vi "HEWH ANSI Display.vi"(5 "Calculation Type":string(combo), 7 "Stop Timer":dbl=1200.0 format="%#_13g", 8 "Error In":errorcluster, 9 "Software Elapsed Time":dbl, 11 "ANSI Rate In":T1) -> (0 "Error Out":errorcluster, 1 "Raw Timer":dbl, 2 "ANSI Display":string, 3 "ANSI Rate Out":T1)   [LabVIEW 2023]
uses:
  HEWH ANSI Rate.ctl
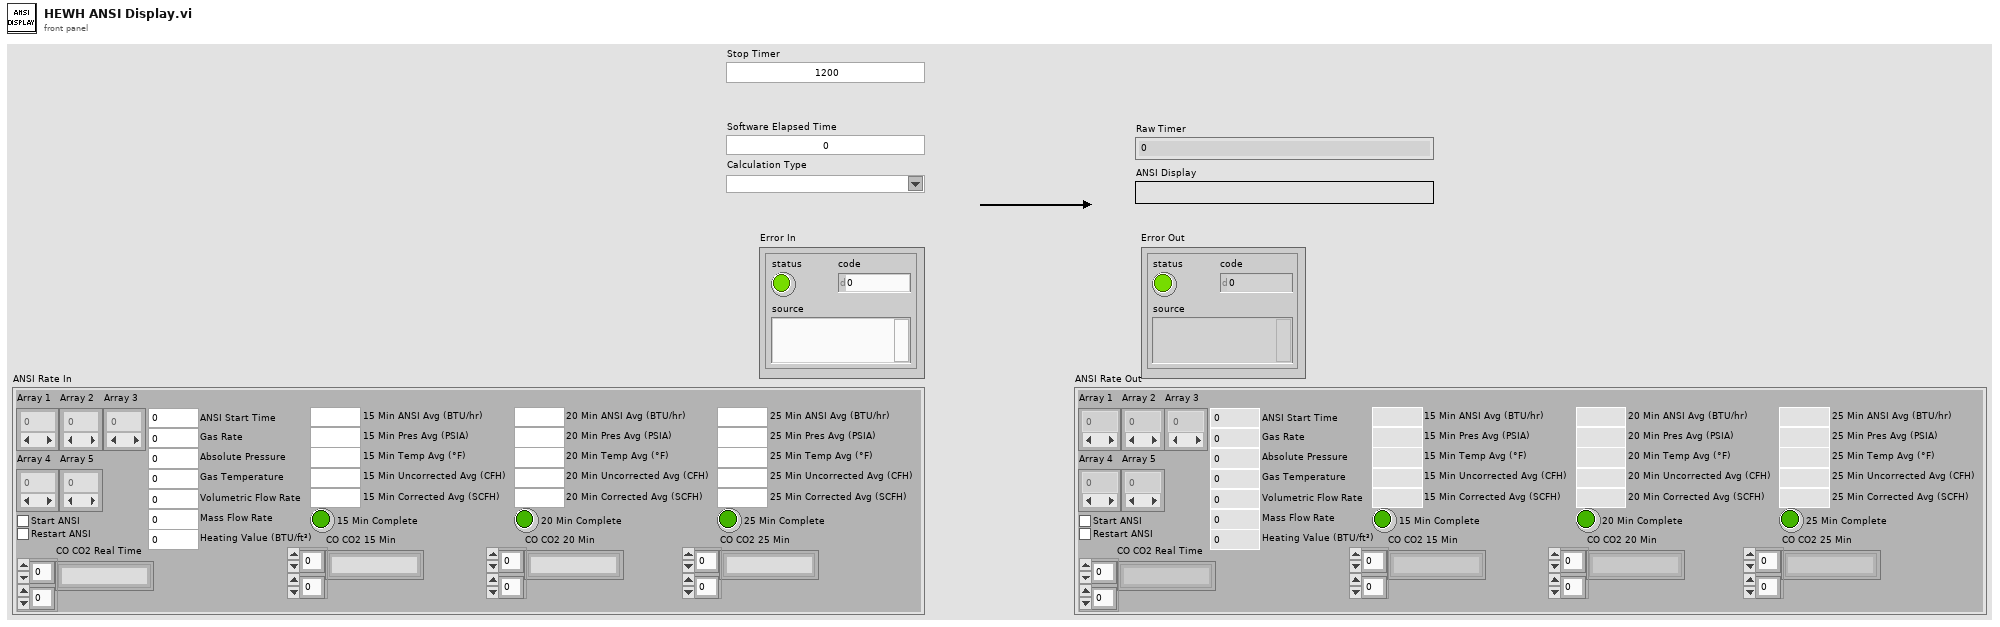
[diagram p1: front panel]
types:
  T1 = typedef "HEWH ANSI Rate.ctl" = cluster{"Array 1":dbl[], "Array 3":dbl[], "Array 2":dbl[], "Start ANSI":bool, "ANSI Start Time":dbl, "Restart ANSI":bool, "15 Min ANSI Avg (BTU/hr)":dbl, "20 Min ANSI Avg (BTU/hr)":dbl, "25 Min ANSI Avg (BTU/hr)":dbl, "Absolute Pressure":dbl, "Gas Temperature":dbl, "Volumetric Flow Rate":dbl, "Mass Flow Rate":dbl, "Array 4":dbl[], "Array 5":dbl[], "Gas Rate":dbl, "15 Min Pres Avg (PSIA)":dbl, "20 Min Pres Avg (PSIA)":dbl, "25 Min Pres Avg (PSIA)":dbl, "15 Min Temp Avg (°F) ":dbl, "20 Min Temp Avg (°F)":dbl, "25 Min Temp Avg (°F)":dbl, "15 Min Uncorrected Avg (CFH)":dbl, "20 Min Uncorrected Avg (CFH)":dbl, "25 Min Uncorrected Avg (CFH)":dbl, "15 Min Corrected Avg (SCFH)":dbl, "20 Min Corrected Avg (SCFH)":dbl, "25 Min Corrected Avg (SCFH)":dbl, "15 Min Complete":bool, "20 Min Complete":bool, "25 Min Complete":bool, "Heating Value (BTU/ft³)":dbl, "CO CO2 15 Min":string[][], "CO CO2 20 Min":string[][], "CO CO2 25 Min":string[][], "CO CO2 Real Time":string[][]}
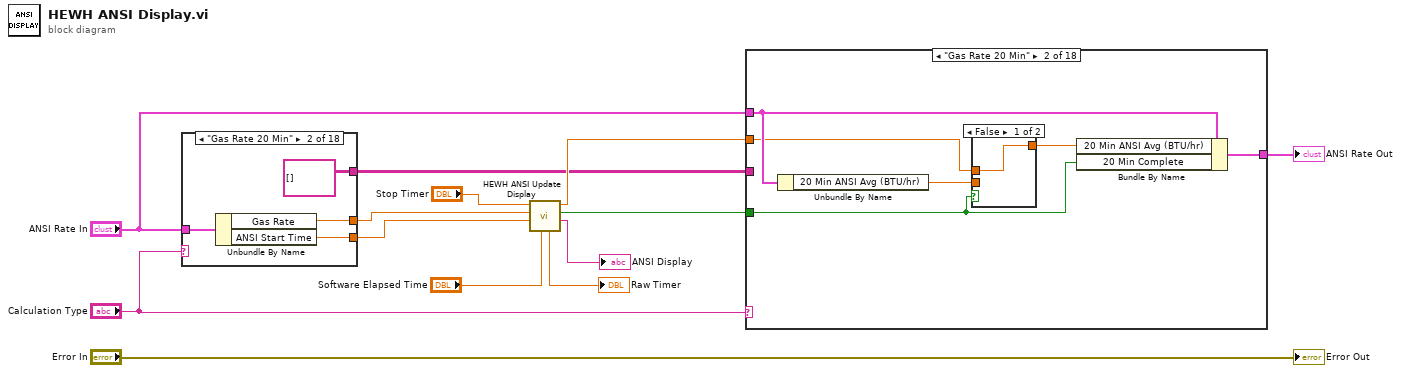
[diagram p0: block diagram]
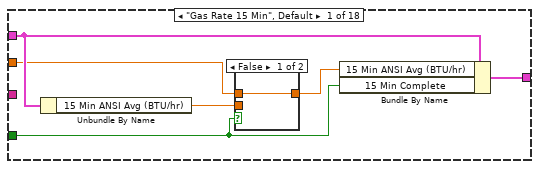
[diagram p2: hidden frame]
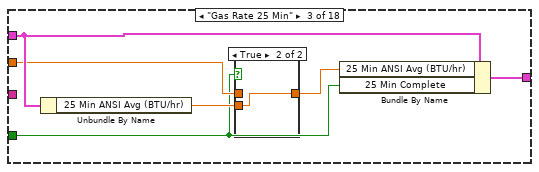
[diagram p5: hidden frame]
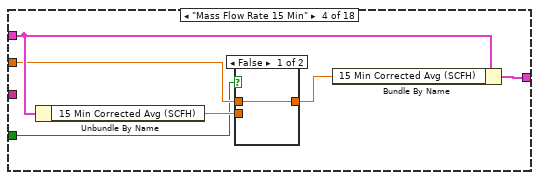
[diagram p7: hidden frame]
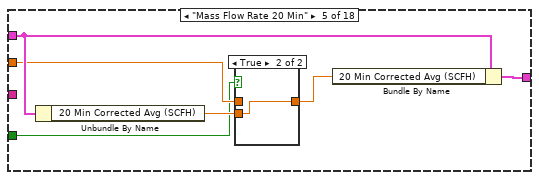
[diagram p9: hidden frame]
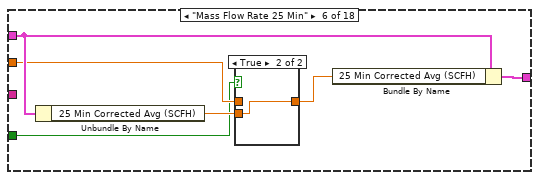
[diagram p11: hidden frame]
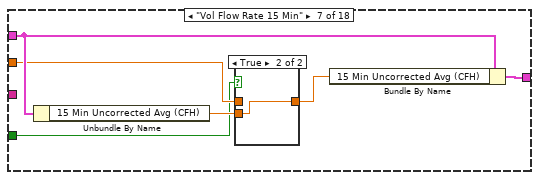
[diagram p13: hidden frame]
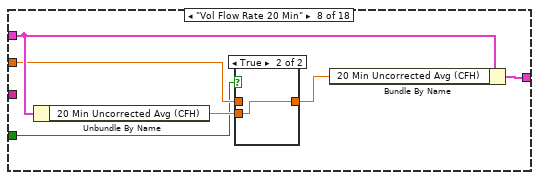
[diagram p15: hidden frame]
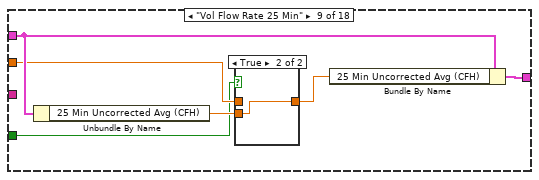
[diagram p17: hidden frame]
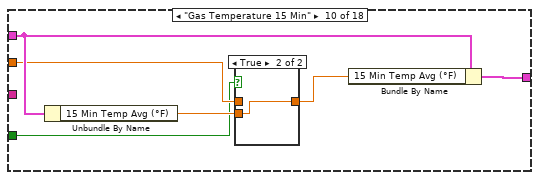
[diagram p19: hidden frame]
diagram:
  n1 = case shown="\"Gas Rate 20 Min\"" "Calculation Type" {
    tunnel: "ANSI Rate In" -> [w17 w21 w25 w29 w33 w37 w41 w45 w49 w53 w57 w61 w65 w69 w73 w77 w81 w85]
    tunnel: [w16 w19 w23 w27 w31 w35 w39 w43 w47 w51 w55 w59 w63 w67 w71 w76 w79 w83] -> w10
    tunnel: [w15 w20 w24 w28 w32 w36 w40 w44 w48 w52 w56 w60 w64 w68 w72 0.0 ("Absolute Pressure") 0.0 ("Absolute Pressure") 0.0 ("Absolute Pressure")] -> w9
    tunnel: [string[][] [] ("CO CO2 25 Min") string[][] [] ("CO CO2 25 Min") string[][] [] ("CO CO2 25 Min") string[][] [] ("CO CO2 25 Min") string[][] [] ("CO CO2 25 Min") string[][] [] ("CO CO2 25 Min") string[][] [] ("CO CO2 25 Min") string[][] [] ("CO CO2 25 Min") string[][] [] ("CO CO2 25 Min") string[][] [] ("CO CO2 25 Min") string[][] [] ("CO CO2 25 Min") string[][] [] ("CO CO2 25 Min") string[][] [] ("CO CO2 25 Min") string[][] [] ("CO CO2 25 Min") string[][] [] ("CO CO2 25 Min") w74 w80 w84] -> w3
    frame "Gas Rate 15 Min", Default {
      n2 = Unbundle By Name(w17) -> ("Gas Rate"=w15:dbl, "ANSI Start Time"=w16:dbl)
    }
    frame "Gas Rate 20 Min" {
      n3 = Unbundle By Name(w21) -> ("Gas Rate"=w20:dbl, "ANSI Start Time"=w19:dbl)
    }
    frame "Gas Rate 25 Min" {
      n4 = Unbundle By Name(w25) -> ("Gas Rate"=w24:dbl, "ANSI Start Time"=w23:dbl)
    }
    frame "Mass Flow Rate 15 Min" {
      n5 = Unbundle By Name(w29) -> ("Mass Flow Rate"=w28:dbl, "ANSI Start Time"=w27:dbl)
    }
    frame "Mass Flow Rate 20 Min" {
      n6 = Unbundle By Name(w33) -> ("Mass Flow Rate"=w32:dbl, "ANSI Start Time"=w31:dbl)
    }
    frame "Mass Flow Rate 25 Min" {
      n7 = Unbundle By Name(w37) -> ("Mass Flow Rate"=w36:dbl, "ANSI Start Time"=w35:dbl)
    }
    frame "Vol Flow Rate 15 Min" {
      n8 = Unbundle By Name(w41) -> ("Volumetric Flow Rate"=w40:dbl, "ANSI Start Time"=w39:dbl)
    }
    frame "Vol Flow Rate 20 Min" {
      n9 = Unbundle By Name(w45) -> ("Volumetric Flow Rate"=w44:dbl, "ANSI Start Time"=w43:dbl)
    }
    frame "Vol Flow Rate 25 Min" {
      n10 = Unbundle By Name(w49) -> ("Volumetric Flow Rate"=w48:dbl, "ANSI Start Time"=w47:dbl)
    }
    frame "Gas Temperature 15 Min" {
      n11 = Unbundle By Name(w53) -> ("Gas Temperature"=w52:dbl, "ANSI Start Time"=w51:dbl)
    }
    frame "Gas Temperature 20 Min" {
      n12 = Unbundle By Name(w57) -> ("Gas Temperature"=w56:dbl, "ANSI Start Time"=w55:dbl)
    }
    frame "Gas Temperature 25 Min" {
      n13 = Unbundle By Name(w61) -> ("Gas Temperature"=w60:dbl, "ANSI Start Time"=w59:dbl)
    }
    frame "Gas Pressure 15 Min" {
      n14 = Unbundle By Name(w65) -> ("Absolute Pressure"=w64:dbl, "ANSI Start Time"=w63:dbl)
    }
    frame "Gas Pressure 20 Min" {
      n15 = Unbundle By Name(w69) -> ("Absolute Pressure"=w68:dbl, "ANSI Start Time"=w67:dbl)
    }
    frame "Gas Pressure 25 Min" {
      n16 = Unbundle By Name(w73) -> ("Absolute Pressure"=w72:dbl, "ANSI Start Time"=w71:dbl)
    }
    frame "CO CO2 15 Min" {
      n17 = Unbundle By Name(w77) -> ("CO CO2 Real Time"=w74:string[][], "ANSI Start Time"=w76:dbl)
    }
    frame "CO CO2 20 Min" {
      n18 = Unbundle By Name(w81) -> ("CO CO2 Real Time"=w80:string[][], "ANSI Start Time"=w79:dbl)
    }
    frame "CO CO2 25 Min" {
      n19 = Unbundle By Name(w85) -> ("CO CO2 Real Time"=w84:string[][], "ANSI Start Time"=w83:dbl)
    }
  }
  n20 = call "HEWH ANSI Update Display.vi"("Software Elapsed Time"="Software Elapsed Time", "ANSI Start Time"=w10, "Absolute Pressure in"=w9, "Stop Timer"="Stop Timer") -> ("ANSI Display"=→"ANSI Display":string, "Complete"=w4:bool, "Absolute Pressure out"=w5:dbl, "Raw Timer"=→"Raw Timer":dbl)  [unwired: 4 in]
  n21 = case shown="\"Gas Rate 20 Min\"" "Calculation Type" {
    tunnel: [w89 w96 w103 w113 w121 w129 w137 w145 w152 w160 w168 w176 w184 w192 w200 w208 w215 w222] -> w8
    tunnel: "ANSI Rate In" -> [w88 w97 w105 w112 w120 w128 w136 w144 w153 w161 w169 w177 w185 w193 w201 w209 w217 w225]
    tunnel: w5 -> [w87 w95 w104 w111 w119 w127 w135 w143 w151 w159 w167 w175 w183 w191 w199 _ _ _]
    tunnel: w4 -> [w86 w94 w102 w110 w118 w126 w134 w142 w150 w158 w166 w174 w182 w190 w198 w206 w214 w223]
    tunnel: w3 -> [_ _ _ _ _ _ _ _ _ _ _ _ _ _ _ w207 w216 w224]
    frame "Gas Rate 15 Min", Default {
      n22 = Unbundle By Name(w88) -> ("15 Min ANSI Avg (BTU/hr)"=w91:dbl)
      n23 = case shown="False" w86 {
        tunnel: w91 -> [_ w93]
        tunnel: [w92 w93] -> w90
        tunnel: w87 -> [w92 _]
        frame False {
        }
        frame True {
        }
      }
      n24 = Bundle By Name(cluster=w88, "15 Min ANSI Avg (BTU/hr)"=w90, "15 Min Complete"=w86) -> (w89:T1)
    }
    frame "Gas Rate 20 Min" {
      n25 = Unbundle By Name(w97) -> ("20 Min ANSI Avg (BTU/hr)"=w99:dbl)
      n26 = case shown="False" w94 {
        tunnel: w99 -> [_ w101]
        tunnel: [w100 w101] -> w98
        tunnel: w95 -> [w100 _]
        frame False {
        }
        frame True {
        }
      }
      n27 = Bundle By Name(cluster=w97, "20 Min ANSI Avg (BTU/hr)"=w98, "20 Min Complete"=w94) -> (w96:T1)
    }
    frame "Gas Rate 25 Min" {
      n28 = Unbundle By Name(w105) -> ("25 Min ANSI Avg (BTU/hr)"=w107:dbl)
      n29 = case shown="True" w102 {
        tunnel: w107 -> [_ w109]
        tunnel: [w108 w109] -> w106
        tunnel: w104 -> [w108 _]
        frame False {
        }
        frame True {
        }
      }
      n30 = Bundle By Name(cluster=w105, "25 Min ANSI Avg (BTU/hr)"=w106, "25 Min Complete"=w102) -> (w103:T1)
    }
    frame "Mass Flow Rate 15 Min" {
      n31 = Unbundle By Name(w112) -> ("15 Min Corrected Avg (SCFH)"=w115:dbl)
      n32 = case shown="False" w110 {
        tunnel: w115 -> [_ w117]
        tunnel: [w116 w117] -> w114
        tunnel: w111 -> [w116 _]
        frame False {
        }
        frame True {
        }
      }
      n33 = Bundle By Name(cluster=w112, "15 Min Corrected Avg (SCFH)"=w114) -> (w113:T1)
    }
    frame "Mass Flow Rate 20 Min" {
      n34 = Unbundle By Name(w120) -> ("20 Min Corrected Avg (SCFH)"=w123:dbl)
      n35 = case shown="True" w118 {
        tunnel: w123 -> [_ w125]
        tunnel: [w124 w125] -> w122
        tunnel: w119 -> [w124 _]
        frame False {
        }
        frame True {
        }
      }
      n36 = Bundle By Name(cluster=w120, "20 Min Corrected Avg (SCFH)"=w122) -> (w121:T1)
    }
    frame "Mass Flow Rate 25 Min" {
      n37 = Unbundle By Name(w128) -> ("25 Min Corrected Avg (SCFH)"=w131:dbl)
      n38 = case shown="True" w126 {
        tunnel: w131 -> [_ w133]
        tunnel: [w132 w133] -> w130
        tunnel: w127 -> [w132 _]
        frame False {
        }
        frame True {
        }
      }
      n39 = Bundle By Name(cluster=w128, "25 Min Corrected Avg (SCFH)"=w130) -> (w129:T1)
    }
    frame "Vol Flow Rate 15 Min" {
      n40 = Unbundle By Name(w136) -> ("15 Min Uncorrected Avg (CFH)"=w139:dbl)
      n41 = case shown="True" w134 {
        tunnel: w139 -> [_ w141]
        tunnel: [w140 w141] -> w138
        tunnel: w135 -> [w140 _]
        frame False {
        }
        frame True {
        }
      }
      n42 = Bundle By Name(cluster=w136, "15 Min Uncorrected Avg (CFH)"=w138) -> (w137:T1)
    }
    frame "Vol Flow Rate 20 Min" {
      n43 = Unbundle By Name(w144) -> ("20 Min Uncorrected Avg (CFH)"=w147:dbl)
      n44 = case shown="True" w142 {
        tunnel: w147 -> [_ w149]
        tunnel: [w148 w149] -> w146
        tunnel: w143 -> [w148 _]
        frame False {
        }
        frame True {
        }
      }
      n45 = Bundle By Name(cluster=w144, "20 Min Uncorrected Avg (CFH)"=w146) -> (w145:T1)
    }
    frame "Vol Flow Rate 25 Min" {
      n46 = Unbundle By Name(w153) -> ("25 Min Uncorrected Avg (CFH)"=w155:dbl)
      n47 = case shown="True" w150 {
        tunnel: w155 -> [_ w157]
        tunnel: [w156 w157] -> w154
        tunnel: w151 -> [w156 _]
        frame False {
        }
        frame True {
        }
      }
      n48 = Bundle By Name(cluster=w153, "25 Min Uncorrected Avg (CFH)"=w154) -> (w152:T1)
    }
    frame "Gas Temperature 15 Min" {
      n49 = Unbundle By Name(w161) -> ("15 Min Temp Avg (°F)"=w163:dbl)
      n50 = case shown="True" w158 {
        tunnel: w163 -> [_ w165]
        tunnel: [w164 w165] -> w162
        tunnel: w159 -> [w164 _]
        frame False {
        }
        frame True {
        }
      }
      n51 = Bundle By Name(cluster=w161, "15 Min Temp Avg (°F)"=w162) -> (w160:T1)
    }
    frame "Gas Temperature 20 Min" {
      n52 = Unbundle By Name(w169) -> ("20 Min Temp Avg (°F)"=w171:dbl)
      n53 = case shown="True" w166 {
        tunnel: w171 -> [_ w173]
        tunnel: [w172 w173] -> w170
        tunnel: w167 -> [w172 _]
        frame False {
        }
        frame True {
        }
      }
      n54 = Bundle By Name(cluster=w169, "20 Min Temp Avg (°F)"=w170) -> (w168:T1)
    }
    frame "Gas Temperature 25 Min" {
      n55 = Unbundle By Name(w177) -> ("25 Min Temp Avg (°F)"=w179:dbl)
      n56 = case shown="True" w174 {
        tunnel: w179 -> [_ w181]
        tunnel: [w180 w181] -> w178
        tunnel: w175 -> [w180 _]
        frame False {
        }
        frame True {
        }
      }
      n57 = Bundle By Name(cluster=w177, "25 Min Temp Avg (°F)"=w178) -> (w176:T1)
    }
    frame "Gas Pressure 15 Min" {
      n58 = Unbundle By Name(w185) -> ("15 Min Pres Avg (PSIA)"=w187:dbl)
      n59 = case shown="True" w182 {
        tunnel: w187 -> [_ w189]
        tunnel: [w188 w189] -> w186
        tunnel: w183 -> [w188 _]
        frame False {
        }
        frame True {
        }
      }
      n60 = Bundle By Name(cluster=w185, "15 Min Pres Avg (PSIA)"=w186) -> (w184:T1)
    }
    frame "Gas Pressure 20 Min" {
      n61 = Unbundle By Name(w193) -> ("20 Min Pres Avg (PSIA)"=w195:dbl)
      n62 = case shown="True" w190 {
        tunnel: w195 -> [_ w197]
        tunnel: [w196 w197] -> w194
        tunnel: w191 -> [w196 _]
        frame False {
        }
        frame True {
        }
      }
      n63 = Bundle By Name(cluster=w193, "20 Min Pres Avg (PSIA)"=w194) -> (w192:T1)
    }
    frame "Gas Pressure 25 Min" {
      n64 = Unbundle By Name(w201) -> ("25 Min Pres Avg (PSIA)"=w203:dbl)
      n65 = case shown="True" w198 {
        tunnel: w203 -> [_ w205]
        tunnel: [w204 w205] -> w202
        tunnel: w199 -> [w204 _]
        frame False {
        }
        frame True {
        }
      }
      n66 = Bundle By Name(cluster=w201, "25 Min Pres Avg (PSIA)"=w202) -> (w200:T1)
    }
    frame "CO CO2 15 Min" {
      n67 = Unbundle By Name(w209) -> ("CO CO2 15 Min"=w211:string[][])
      n68 = case shown="True" w206 {
        tunnel: w211 -> [_ w213]
        tunnel: [w212 w213] -> w210
        tunnel: w207 -> [w212 _]
        frame False {
        }
        frame True {
        }
      }
      n69 = Bundle By Name(cluster=w209, "CO CO2 15 Min"=w210) -> (w208:T1)
    }
    frame "CO CO2 20 Min" {
      n70 = Unbundle By Name(w217) -> ("CO CO2 20 Min"=w219:string[][])
      n71 = case shown="False" w214 {
        tunnel: w219 -> [_ w221]
        tunnel: [w220 w221] -> w218
        tunnel: w216 -> [w220 _]
        frame False {
        }
        frame True {
        }
      }
      n72 = Bundle By Name(cluster=w217, "CO CO2 20 Min"=w218) -> (w215:T1)
    }
    frame "CO CO2 25 Min" {
      n73 = Unbundle By Name(w225) -> ("CO CO2 25 Min"=w227:string[][])
      n74 = case shown="False" w223 {
        tunnel: w227 -> [_ w229]
        tunnel: [w228 w229] -> w226
        tunnel: w224 -> [w228 _]
        frame False {
        }
        frame True {
        }
      }
      n75 = Bundle By Name(cluster=w225, "CO CO2 25 Min"=w226) -> (w222:T1)
    }
  }
  "ANSI Rate Out" <- w8
  "Error Out" <- "Error In"
